vi "All together marble sorter code - working version 4_15.vi"() -> ()   [LabVIEW 2016]
uses:
  <vilib>/NXT/Block Support/NXT_InputPort.ctl
  <vilib>/NXT/Block Support/NXT_OutputPort.ctl
  <vilib>/NXT/Dual Mode Library/Sensors/Touch_Bumped.vi
  <vilib>/NXT/NXTIO Xnodes/NXTIONodeSubVIs/NXTMotorRunDistance.vi
  <vilib>/NXT/NXTIO Xnodes/NXTIONodeSubVIs/LEGOMoveAllMotorsDistance.vi
  <vilib>/NXT/Dual Mode Library/Sensors/Touch_Count.vi
  <vilib>/NXT/Dual Mode Library/Sensors/EV3_Color_Reflect.vi
  <vilib>/NXT/NXTIO Xnodes/NXTIONodeSubVIs/NXTStopMotors.vi
  <vilib>/NXT/NXTIO Xnodes/AddressXNode/NXTIOAddress.xnode
  <vilib>/NXT/NXTIO Xnodes/NXTIOXNode/NXTIO.xnode
  <vilib>/NXT/Subs/LVHSConnector.ctl
  <vilib>/NXT/LegoClasses/BrickReference/BrickReference.lvclass
panel:
  out "Marble Type 5":string
  out "Type 1 count 4":string
  out "Type 2 Count 4":string
  out "Marble Type 4 Code":i32[](array[numeric])
  out "Marble Count 4 Code":i32[](array[numeric])
  out "Marble Type 4":string
  out "Type 1 Count 3":string
  out "Type 2 Count 3":string
  out "Marble Count 3":i32[](array[numeric])
  out "Marble Type 3":i32[](array[numeric])
  out "Marble Type 2":string
  out "Type 1 Count 2":string
  out "Type 2 Count 2":string
  out "Marble Count 2 Code":i32[](array[numeric])
  out "Marble Type 2 Code":i32[](array[numeric])
  out "Marble Type code":i32[](array[numeric])
  out "Marble Size code":i32[](array[numeric])
  out "Marble Type":string
  out "Type 2 Count":string
  out "Type 1 Count":string
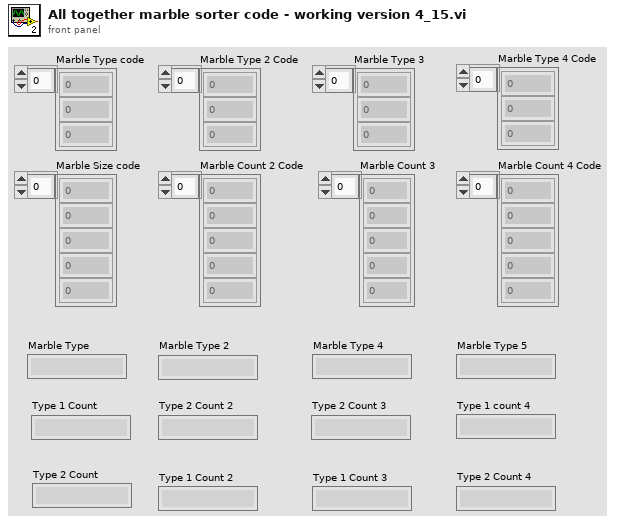
[diagram p1: front panel]
types:
  T1 = typedef "NXT_InputPort.ctl" = u32
  T2 = typedef "LVHSConnector.ctl" = refnum<class "BrickReference.lvclass">
  T3 = typedef "NXT_OutputPort.ctl" = u8
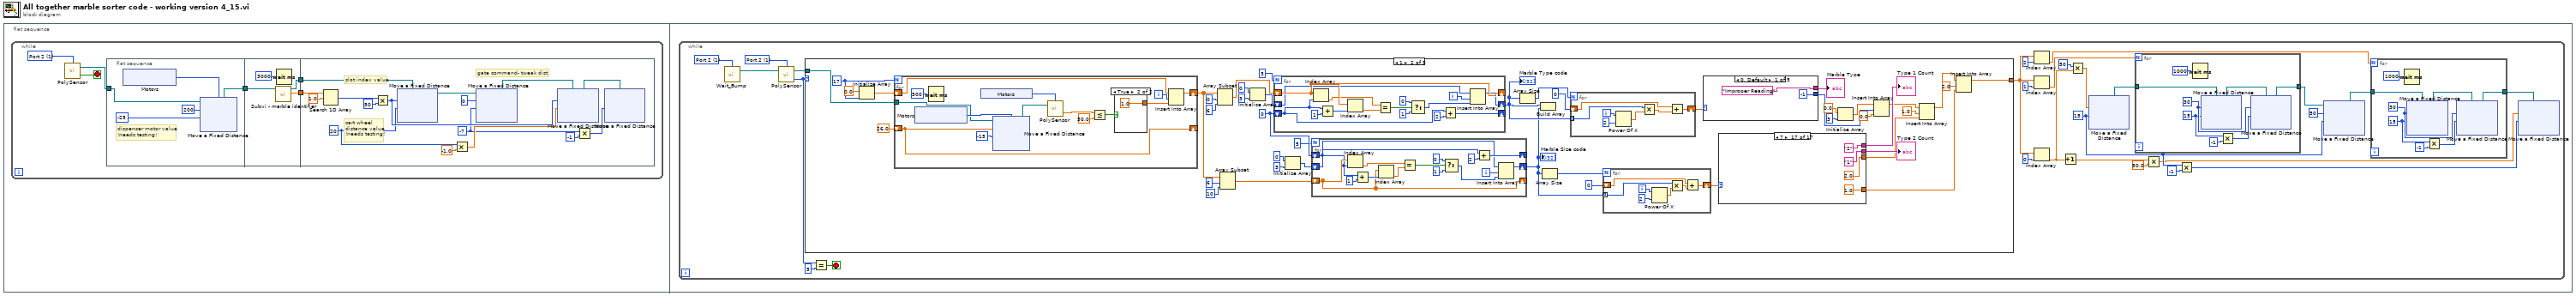
[diagram p0: block diagram]
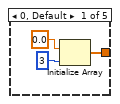
[diagram p2: hidden frame]
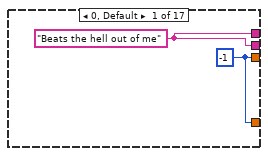
[diagram p3: hidden frame]
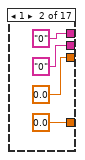
[diagram p4: hidden frame]
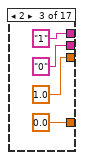
[diagram p5: hidden frame]
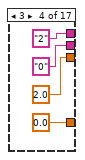
[diagram p6: hidden frame]
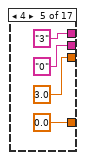
[diagram p7: hidden frame]
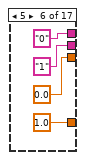
[diagram p8: hidden frame]
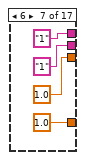
[diagram p9: hidden frame]
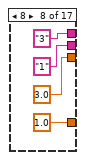
[diagram p10: hidden frame]
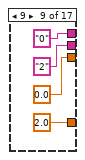
[diagram p11: hidden frame]
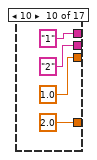
[diagram p12: hidden frame]
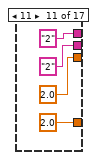
[diagram p13: hidden frame]
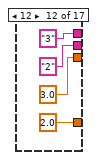
[diagram p14: hidden frame]
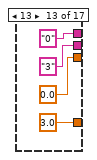
[diagram p15: hidden frame]
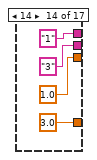
[diagram p16: hidden frame]
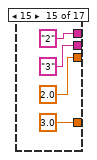
[diagram p17: hidden frame]
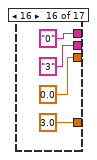
[diagram p18: hidden frame]
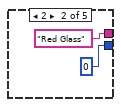
[diagram p19: hidden frame]
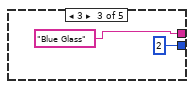
[diagram p20: hidden frame]
diagram:
  n1 = flat-sequence {
    frame #0 {
      n2 = while {
        stop <- w3 stop-if-true
        w1 = T1 1 items=["Port 1", "Port 2", "Port 3", "Port 4"] ("Port (Port 1)")
        n3 = call-poly <vilib>:"PolySensor.vi"("Port (Port 1)"=w1) -> ("Yes / No"=w3:bool, "NXT/EV3"=w2:T2)  [unwired: 2 in]
        n4 = flat-sequence {
          tunnel: [w8] -> w5
          tunnel: w2 -> [w7]
          tunnel: [w25] -> w6
          tunnel: w5 -> [w26]
          tunnel: [w24] -> w4
          tunnel: w6 -> [w37]
          tunnel: w4 -> [w28]
          frame #0 {
            # "dispenser motor value\n!needs testing!"
            n5 = xnode "Motors"() -> ("Motor"=w11:T3)
            n6 = xnode "Move a Fixed Distance"("Speed 1"=-25, "Distance 1"=200, "Motors"=w11, "NXT/EV3"=w7) -> ("NXT/EV3"=w8:T2)
          }
          frame #1 {
            n7 = call "Subvi - marble identifier.vi"("BrickReference in"=w26) -> ("Array"=w24:dbl[], "BrickReference out"=w25:T2)  [unwired: 9 in]
            n8 = Wait (ms)(milliseconds to wait=u32 3000) -> ()  [unwired: 1 out]
          }
          frame #2 {
            w30 = i8 -7 ("Speed 1")
            w39 = i8 20 ("Speed 1")
            # "gate command- tweak dist"
            # "cart wheel\ndistance value\n!needs testing!"
            # "slot index value"
            n9 = Search 1D Array(1D array=w28, element=1.0) -> (index of element=w27:i32)  [unwired: 1 in]
            n10 = Multiply(x=w27, y=50) -> (x*y=w41:i32)
            n11 = xnode "Move a Fixed Distance"("Speed 1"=w39, "Distance 1"=w41, "NXT/EV3"=w37) -> ("NXT/EV3"=w36:T2)  [unwired: 1 in]
            n12 = Multiply(x=w39, y=-1.0) -> (x*y=w38:dbl)
            n13 = xnode "Move a Fixed Distance"("Speed 1"=w30, "Distance 1"=0, "NXT/EV3"=w36) -> ("NXT/EV3"=w35:T2)  [unwired: 1 in]
            n14 = xnode "Move a Fixed Distance"("Speed 1"=w38, "Distance 1"=w41, "NXT/EV3"=w35) -> ("NXT/EV3"=w34:T2)  [unwired: 1 in]
            n15 = Multiply(x=w30, y=-1) -> (x*y=w31:i32)
            n16 = xnode "Move a Fixed Distance"("Speed 1"=w31, "NXT/EV3"=w34) -> ()  [unwired: 2 in, 1 out]
          }
        }
      }
    }
    frame #1 {
      n17 = while {
        stop <- w92 stop-if-true
        w77 = i8 15 ("Speed 1")
        w94 = T1 1 items=["Port 1", "Port 2", "Port 3", "Port 4"] ("Port (Port 1)")
        w95 = T1 1 items=["Port 1", "Port 2", "Port 3", "Port 4"] ("Port (Port 1)")
        n18 = call <vilib>:"Wait_Bump.vi"("Port (Port 1)"=w95) -> ("NXT/EV3"=w97:T2)  [unwired: 3 in]
        n19 = call-poly <vilib>:"PolySensor.vi"("NXT/EV3"=w97, "Port (Port 1)"=w94) -> ("Count"=w91:i16, "NXT/EV3"=w96:T2)  [unwired: 1 in]
        n20 = case shown="1" w91 {
          tunnel: w96 -> [_ w178 w375 w567 w766]
          tunnel: [w163 w166 w358 w550 w749] -> w81
          frame 0, Default {
            n21 = Initialize Array(0.0 ("element"), 3 ("dimension size")) -> (w163:dbl[])
          }
          frame 1 {
            w192 = 0
            w209 = 17
            n22 = Initialize Array(0.0, w209) -> (w207:dbl[])
            n23 = for {
              N: w209 -> [_]
              shift-right: [w338] -> w184
              shift-left: w207 -> [w342]
              shift-right: [w335] -> _
              shift-left: 26.0 -> [w335]
              tunnel: w178 -> [w330]
              i -> [w343]
              n24 = xnode "Motors"() -> ("Motor"=w333:T3)
              n25 = Wait (ms)(milliseconds to wait=500) -> ()  [unwired: 1 out]
              n26 = xnode "Motors"() -> ("Sensor"=w337:T1)
              n27 = xnode "Move a Fixed Distance"("Speed 1"=i8 -15, "Distance 1"=w335, "Motors"=w333, "NXT/EV3"=w330) -> ("NXT/EV3"=w334:T2)
              n28 = call-poly <vilib>:"PolySensor.vi"("NXT/EV3"=w334, "Port (Port 1)"=w337) -> ("Scaled Value"=w336:sgl)  [unwired: 1 in, 1 out]
              n29 = Less Or Equal?(x=w336, y=50.0) -> (x <= y?=w340:bool)
              n30 = case shown="True" w340 {
                tunnel: [0.0 1.0] -> w339
                frame False {
                }
                frame True {
                }
              }
              n31 = Insert Into Array(array=w342, index=w343, new element=w339) -> (w338:dbl[])
            }
            n32 = Array Subset(array=w184, index=0, length=6) -> (w200:dbl[])
            n33 = Array Subset(array=w184, index=6, length=10) -> (w196:dbl[])
            n34 = Initialize Array(0, 3 ("dimension size")) -> (w198:i32[])
            n35 = for {
              N: 3 -> [_]
              shift-right: [w327] -> _
              shift-left: w200 -> [w327]
              shift-right: [w319] -> _
              shift-left: w192 -> [w320]
              shift-right: [w317] -> w183
              shift-left: w198 -> [w316]
              i -> [w315]
              n36 = Index Array(array=w327, index=w320) -> (element=w324:dbl)
              n37 = Add(x=w320, y=1) -> (x+y=w328:i32)
              n38 = Index Array(array=w327, index=w328) -> (element=w323:dbl)
              n39 = Equal?(x=w324, y=w323) -> (x = y?=w322:bool)
              n40 = Select(t=0, s=w322, f=1) -> (s? t:f=w321:i32)
              n41 = Add(x=w320, y=2) -> (x+y=w319:i32)
              n42 = Insert Into Array(array=w316, index=w315, new element=w321) -> (w317:i32[])
            }
            "Marble Type code" <- w183
            n43 = Initialize Array(0, 5 ("dimension size")) -> (w193:i32[])
            n44 = for {
              N: 5 -> [_]
              shift-right: [w312] -> _
              shift-left: w196 -> [w312]
              shift-right: [w304] -> _
              shift-left: w192 -> [w305]
              shift-right: [w302] -> w182
              shift-left: w193 -> [w301]
              i -> [w300]
              n45 = Index Array(array=w312, index=w305) -> (element=w309:dbl)
              n46 = Add(x=w305, y=1) -> (x+y=w313:i32)
              n47 = Index Array(array=w312, index=w313) -> (element=w308:dbl)
              n48 = Equal?(x=w309, y=w308) -> (x = y?=w307:bool)
              n49 = Select(t=0, s=w307, f=1) -> (s? t:f=w306:i32)
              n50 = Add(x=w305, y=2) -> (x+y=w304:i32)
              n51 = Insert Into Array(array=w301, index=w300, new element=w306) -> (w302:i32[])
            }
            "Marble Size code" <- w182
            n52 = Array Size(array=w183) -> (size(s)=w190:i32)
            n53 = Build Array(w183, w182) -> ()  [unwired: 1 out]
            n54 = Array Size(array=w182) -> (size(s)=w187:i32)
            n55 = for {
              N: w190 -> [_]
              tunnel: w183 -> [w220] mode=indexing
              shift-right: [w217] -> w188
              shift-left: 0 -> [w218]
              i -> [w222]
              n56 = Power Of X(1:2, 2:w222) -> (0:w221:dbl)
              n57 = Multiply(x=w220, y=w221) -> (x*y=w219:dbl)
              n58 = Add(x=w218, y=w219) -> (x+y=w217:dbl)
            }
            n59 = for {
              N: w187 -> [_]
              tunnel: w182 -> [w213] mode=indexing
              shift-right: [w210] -> w185
              shift-left: 0 -> [w211]
              i -> [w215]
              n60 = Power Of X(1:2, 2:w215) -> (0:w214:dbl)
              n61 = Multiply(x=w213, y=w214) -> (x*y=w212:dbl)
              n62 = Add(x=w211, y=w212) -> (x+y=w210:dbl)
            }
            n63 = case shown="0, Default" w188 {
              tunnel: ["Improper Reading" "Red Glass" "Blue Glass" "White Glass" "Steel/HDPE"] -> w179
              tunnel: [-1 0 2 4 6] -> w169
              frame 0, Default {
              }
              frame 2 {
              }
              frame 3 {
              }
              frame 1 {
              }
              frame 4 {
              }
            }
            "Marble Type" <- w179
            n64 = case shown="7" w185 {
              tunnel: [w225 "0" "1" "2" "3" "0" "1" "3" "0" "1" "2" "3" "0" "1" "2" "0" "2"] -> w181
              tunnel: [w225 "0" "0" "0" "0" "1" "1" "1" "2" "2" "2" "2" "3" "3" "3" "3" "1"] -> w180
              tunnel: [w224 0.0 ("new element/subarray") 1.0 ("new element/subarray") 2.0 ("new element/subarray") 3.0 ("new element/subarray") 0.0 ("new element/subarray") 1.0 ("new element/subarray") 3.0 ("new element/subarray") 0.0 ("new element/subarray") 1.0 ("new element/subarray") 2.0 ("new element/subarray") 3.0 ("new element/subarray") 0.0 ("new element/subarray") 1.0 ("new element/subarray") 2.0 ("new element/subarray") 0.0 ("new element/subarray") 2.0 ("new element/subarray")] -> w168
              tunnel: [w224 0.0 ("new element/subarray") 0.0 ("new element/subarray") 0.0 ("new element/subarray") 0.0 ("new element/subarray") 1.0 ("new element/subarray") 1.0 ("new element/subarray") 1.0 ("new element/subarray") 2.0 ("new element/subarray") 2.0 ("new element/subarray") 2.0 ("new element/subarray") 2.0 ("new element/subarray") 3.0 ("new element/subarray") 3.0 ("new element/subarray") 3.0 ("new element/subarray") 3.0 ("new element/subarray") 1.0 ("new element/subarray")] -> w167
              frame 0, Default {
                w224 = -1
                w225 = "Beats the hell out of me"
              }
              frame 1 {
              }
              frame 2 {
              }
              frame 3 {
              }
              frame 4 {
              }
              frame 5 {
              }
              frame 6 {
              }
              frame 8 {
              }
              frame 9 {
              }
              frame 10 {
              }
              frame 11 {
              }
              frame 12 {
              }
              frame 13 {
              }
              frame 14 {
              }
              frame 15 {
              }
              frame 16 {
              }
              frame 7 {
              }
            }
            "Type 2 Count" <- w180
            "Type 1 Count" <- w181
            n65 = Initialize Array(0.0 ("element"), 3 ("dimension size")) -> (w175:dbl[])
            n66 = Insert Into Array(array=w175, index=w169, new element=0.0 ("new element/subarray")) -> (w174:dbl[])
            n67 = Insert Into Array(array=w174, index=1.0 ("new element/subarray"), new element=w168) -> (w173:dbl[])
            n68 = Insert Into Array(array=w173, index=2.0 ("new element/subarray"), new element=w167) -> (w166:dbl[])
          }
          frame 2 {
            w384 = 0
            w401 = 17
            n69 = Initialize Array(0.0, w401) -> (w399:dbl[])
            n70 = for {
              N: w401 -> [_]
              shift-right: [w530] -> w378
              shift-left: w399 -> [w534]
              shift-right: [w527] -> _
              shift-left: 26.0 -> [w527]
              tunnel: w375 -> [w522]
              i -> [w535]
              n71 = xnode "Motors"() -> ("Motor"=w525:T3)
              n72 = Wait (ms)(milliseconds to wait=500) -> ()  [unwired: 1 out]
              n73 = xnode "Motors"() -> ("Sensor"=w529:T1)
              n74 = xnode "Move a Fixed Distance"("Speed 1"=i8 -15, "Distance 1"=w527, "Motors"=w525, "NXT/EV3"=w522) -> ("NXT/EV3"=w526:T2)
              n75 = call-poly <vilib>:"PolySensor.vi"("NXT/EV3"=w526, "Port (Port 1)"=w529) -> ("Scaled Value"=w528:sgl)  [unwired: 1 in, 1 out]
              n76 = Less Or Equal?(x=w528, y=50.0) -> (x <= y?=w532:bool)
              n77 = case shown="True" w532 {
                tunnel: [0.0 1.0] -> w531
                frame False {
                }
                frame True {
                }
              }
              n78 = Insert Into Array(array=w534, index=w535, new element=w531) -> (w530:dbl[])
            }
            n79 = Array Subset(array=w378, index=0, length=6) -> (w392:dbl[])
            n80 = Array Subset(array=w378, index=6, length=10) -> (w388:dbl[])
            n81 = Initialize Array(0, 3 ("dimension size")) -> (w390:i32[])
            n82 = for {
              N: 3 -> [_]
              shift-right: [w519] -> _
              shift-left: w392 -> [w519]
              shift-right: [w511] -> _
              shift-left: w384 -> [w512]
              shift-right: [w509] -> w377
              shift-left: w390 -> [w508]
              i -> [w507]
              n83 = Index Array(array=w519, index=w512) -> (element=w516:dbl)
              n84 = Add(x=w512, y=1) -> (x+y=w520:i32)
              n85 = Index Array(array=w519, index=w520) -> (element=w515:dbl)
              n86 = Equal?(x=w516, y=w515) -> (x = y?=w514:bool)
              n87 = Select(t=0, s=w514, f=1) -> (s? t:f=w513:i32)
              n88 = Add(x=w512, y=2) -> (x+y=w511:i32)
              n89 = Insert Into Array(array=w508, index=w507, new element=w513) -> (w509:i32[])
            }
            "Marble Type 2 Code" <- w377
            n90 = Initialize Array(0, 5 ("dimension size")) -> (w385:i32[])
            n91 = for {
              N: 5 -> [_]
              shift-right: [w504] -> _
              shift-left: w388 -> [w504]
              shift-right: [w496] -> _
              shift-left: w384 -> [w497]
              shift-right: [w494] -> w376
              shift-left: w385 -> [w493]
              i -> [w492]
              n92 = Index Array(array=w504, index=w497) -> (element=w501:dbl)
              n93 = Add(x=w497, y=1) -> (x+y=w505:i32)
              n94 = Index Array(array=w504, index=w505) -> (element=w500:dbl)
              n95 = Equal?(x=w501, y=w500) -> (x = y?=w499:bool)
              n96 = Select(t=0, s=w499, f=1) -> (s? t:f=w498:i32)
              n97 = Add(x=w497, y=2) -> (x+y=w496:i32)
              n98 = Insert Into Array(array=w493, index=w492, new element=w498) -> (w494:i32[])
            }
            "Marble Count 2 Code" <- w376
            n99 = Array Size(array=w377) -> (size(s)=w382:i32)
            n100 = Array Size(array=w376) -> (size(s)=w380:i32)
            n101 = for {
              N: w382 -> [_]
              tunnel: w377 -> [w488] mode=indexing
              shift-right: [w485] -> w361
              shift-left: 0 -> [w486]
              i -> [w490]
              n102 = Power Of X(1:2, 2:w490) -> (0:w489:dbl)
              n103 = Multiply(x=w488, y=w489) -> (x*y=w487:dbl)
              n104 = Add(x=w486, y=w487) -> (x+y=w485:dbl)
            }
            n105 = for {
              N: w380 -> [_]
              tunnel: w376 -> [w481] mode=indexing
              shift-right: [w478] -> w359
              shift-left: 0 -> [w479]
              i -> [w483]
              n106 = Power Of X(1:2, 2:w483) -> (0:w482:dbl)
              n107 = Multiply(x=w481, y=w482) -> (x*y=w480:dbl)
              n108 = Add(x=w479, y=w480) -> (x+y=w478:dbl)
            }
            n109 = case shown="0, Default" w361 {
              tunnel: ["Improper Reading" "Red Glass" "Blue Glass" "White Glass" "Steel/HDPE"] -> w362
              tunnel: [-1 0 2 4 6] -> w360
              frame 0, Default {
              }
              frame 2 {
              }
              frame 3 {
              }
              frame 1 {
              }
              frame 4 {
              }
            }
            "Marble Type 2" <- w362
            n110 = case shown="7" w359 {
              tunnel: [w403 "0" "1" "2" "3" "0" "1" "3" "0" "1" "2" "3" "0" "1" "2" "0" "2"] -> w364
              tunnel: [w403 "0" "0" "0" "0" "1" "1" "1" "2" "2" "2" "2" "3" "3" "3" "3" "1"] -> w363
              tunnel: [w402 0.0 ("new element/subarray") 1.0 ("new element/subarray") 2.0 ("new element/subarray") 3.0 ("new element/subarray") 0.0 ("new element/subarray") 1.0 ("new element/subarray") 3.0 ("new element/subarray") 0.0 ("new element/subarray") 1.0 ("new element/subarray") 2.0 ("new element/subarray") 3.0 ("new element/subarray") 0.0 ("new element/subarray") 1.0 ("new element/subarray") 2.0 ("new element/subarray") 0.0 ("new element/subarray") 2.0 ("new element/subarray")] -> w366
              tunnel: [w402 0.0 ("new element/subarray") 0.0 ("new element/subarray") 0.0 ("new element/subarray") 0.0 ("new element/subarray") 1.0 ("new element/subarray") 1.0 ("new element/subarray") 1.0 ("new element/subarray") 2.0 ("new element/subarray") 2.0 ("new element/subarray") 2.0 ("new element/subarray") 2.0 ("new element/subarray") 3.0 ("new element/subarray") 3.0 ("new element/subarray") 3.0 ("new element/subarray") 3.0 ("new element/subarray") 1.0 ("new element/subarray")] -> w365
              frame 0, Default {
                w402 = -1
                w403 = "Beats the hell out of me"
              }
              frame 1 {
              }
              frame 2 {
              }
              frame 3 {
              }
              frame 4 {
              }
              frame 5 {
              }
              frame 6 {
              }
              frame 8 {
              }
              frame 9 {
              }
              frame 10 {
              }
              frame 11 {
              }
              frame 12 {
              }
              frame 13 {
              }
              frame 14 {
              }
              frame 15 {
              }
              frame 16 {
              }
              frame 7 {
              }
            }
            "Type 1 Count 2" <- w364
            "Type 2 Count 2" <- w363
            n111 = Initialize Array(0.0 ("element"), 3 ("dimension size")) -> (w372:dbl[])
            n112 = Insert Into Array(array=w372, index=w360, new element=0.0 ("new element/subarray")) -> (w371:dbl[])
            n113 = Insert Into Array(array=w371, index=1.0 ("new element/subarray"), new element=w366) -> (w370:dbl[])
            n114 = Insert Into Array(array=w370, index=2.0 ("new element/subarray"), new element=w365) -> (w358:dbl[])
          }
          frame 3 {
            w586 = 0
            w569 = 17
            n115 = Initialize Array(0.0, w569) -> (w571:dbl[])
            n116 = for {
              N: w569 -> [_]
              shift-right: [w723] -> w592
              shift-left: w571 -> [w727]
              shift-right: [w720] -> _
              shift-left: 26.0 -> [w720]
              tunnel: w567 -> [w714]
              i -> [w728]
              n117 = xnode "Motors"() -> ("Motor"=w715:T3)
              n118 = xnode "Motors"() -> ("Motor"=w718:T3)
              n119 = Wait (ms)(milliseconds to wait=500) -> ()  [unwired: 1 out]
              n120 = xnode "Stop Motors"("Motors"=w715) -> ()  [unwired: 1 in, 1 out]
              n121 = xnode "Motors"() -> ("Sensor"=w722:T1)
              n122 = xnode "Move a Fixed Distance"("Speed 1"=i8 -15, "Distance 1"=w720, "Motors"=w718, "NXT/EV3"=w714) -> ("NXT/EV3"=w719:T2)
              n123 = call-poly <vilib>:"PolySensor.vi"("NXT/EV3"=w719, "Port (Port 1)"=w722) -> ("Scaled Value"=w721:sgl)  [unwired: 1 in, 1 out]
              n124 = Less Or Equal?(x=w721, y=50.0) -> (x <= y?=w725:bool)
              n125 = case shown="True" w725 {
                tunnel: [0.0 1.0] -> w724
                frame False {
                }
                frame True {
                }
              }
              n126 = Insert Into Array(array=w727, index=w728, new element=w724) -> (w723:dbl[])
            }
            n127 = Array Subset(array=w592, index=0, length=6) -> (w578:dbl[])
            n128 = Array Subset(array=w592, index=6, length=10) -> (w582:dbl[])
            n129 = Initialize Array(0, 3 ("dimension size")) -> (w580:i32[])
            n130 = for {
              N: 3 -> [_]
              shift-right: [w711] -> _
              shift-left: w578 -> [w711]
              shift-right: [w703] -> _
              shift-left: w586 -> [w704]
              shift-right: [w701] -> w593
              shift-left: w580 -> [w700]
              i -> [w699]
              n131 = Index Array(array=w711, index=w704) -> (element=w708:dbl)
              n132 = Add(x=w704, y=1) -> (x+y=w712:i32)
              n133 = Index Array(array=w711, index=w712) -> (element=w707:dbl)
              n134 = Equal?(x=w708, y=w707) -> (x = y?=w706:bool)
              n135 = Select(t=0, s=w706, f=1) -> (s? t:f=w705:i32)
              n136 = Add(x=w704, y=2) -> (x+y=w703:i32)
              n137 = Insert Into Array(array=w700, index=w699, new element=w705) -> (w701:i32[])
            }
            "Marble Type 3" <- w593
            n138 = Initialize Array(0, 5 ("dimension size")) -> (w585:i32[])
            n139 = for {
              N: 5 -> [_]
              shift-right: [w696] -> _
              shift-left: w582 -> [w696]
              shift-right: [w688] -> _
              shift-left: w586 -> [w689]
              shift-right: [w686] -> w568
              shift-left: w585 -> [w685]
              i -> [w684]
              n140 = Index Array(array=w696, index=w689) -> (element=w693:dbl)
              n141 = Add(x=w689, y=1) -> (x+y=w697:i32)
              n142 = Index Array(array=w696, index=w697) -> (element=w692:dbl)
              n143 = Equal?(x=w693, y=w692) -> (x = y?=w691:bool)
              n144 = Select(t=0, s=w691, f=1) -> (s? t:f=w690:i32)
              n145 = Add(x=w689, y=2) -> (x+y=w688:i32)
              n146 = Insert Into Array(array=w685, index=w684, new element=w690) -> (w686:i32[])
            }
            "Marble Count 3" <- w568
            n147 = Array Size(array=w593) -> (size(s)=w588:i32)
            n148 = Array Size(array=w568) -> (size(s)=w590:i32)
            n149 = for {
              N: w588 -> [_]
              tunnel: w593 -> [w680] mode=indexing
              shift-right: [w677] -> w551
              shift-left: 0 -> [w678]
              i -> [w682]
              n150 = Power Of X(1:2, 2:w682) -> (0:w681:dbl)
              n151 = Multiply(x=w680, y=w681) -> (x*y=w679:dbl)
              n152 = Add(x=w678, y=w679) -> (x+y=w677:dbl)
            }
            n153 = for {
              N: w590 -> [_]
              tunnel: w568 -> [w673] mode=indexing
              shift-right: [w670] -> w552
              shift-left: 0 -> [w671]
              i -> [w675]
              n154 = Power Of X(1:2, 2:w675) -> (0:w674:dbl)
              n155 = Multiply(x=w673, y=w674) -> (x*y=w672:dbl)
              n156 = Add(x=w671, y=w672) -> (x+y=w670:dbl)
            }
            n157 = case shown="0, Default" w551 {
              tunnel: ["Improper Reading" "Red Glass" "Blue Glass" "White Glass" "Steel/HDPE"] -> w556
              tunnel: [-1 0 2 4 6] -> w553
              frame 0, Default {
              }
              frame 2 {
              }
              frame 3 {
              }
              frame 1 {
              }
              frame 4 {
              }
            }
            "Marble Type 4" <- w556
            n158 = case shown="7" w552 {
              tunnel: [w595 "0" "1" "2" "3" "0" "1" "3" "0" "1" "2" "3" "0" "1" "2" "0" "2"] -> w555
              tunnel: [w595 "0" "0" "0" "0" "1" "1" "1" "2" "2" "2" "2" "3" "3" "3" "3" "1"] -> w554
              tunnel: [w594 0.0 ("new element/subarray") 1.0 ("new element/subarray") 2.0 ("new element/subarray") 3.0 ("new element/subarray") 0.0 ("new element/subarray") 1.0 ("new element/subarray") 3.0 ("new element/subarray") 0.0 ("new element/subarray") 1.0 ("new element/subarray") 2.0 ("new element/subarray") 3.0 ("new element/subarray") 0.0 ("new element/subarray") 1.0 ("new element/subarray") 2.0 ("new element/subarray") 0.0 ("new element/subarray") 2.0 ("new element/subarray")] -> w558
              tunnel: [w594 0.0 ("new element/subarray") 0.0 ("new element/subarray") 0.0 ("new element/subarray") 0.0 ("new element/subarray") 1.0 ("new element/subarray") 1.0 ("new element/subarray") 1.0 ("new element/subarray") 2.0 ("new element/subarray") 2.0 ("new element/subarray") 2.0 ("new element/subarray") 2.0 ("new element/subarray") 3.0 ("new element/subarray") 3.0 ("new element/subarray") 3.0 ("new element/subarray") 3.0 ("new element/subarray") 1.0 ("new element/subarray")] -> w557
              frame 0, Default {
                w594 = -1
                w595 = "Beats the hell out of me"
              }
              frame 1 {
              }
              frame 2 {
              }
              frame 3 {
              }
              frame 4 {
              }
              frame 5 {
              }
              frame 6 {
              }
              frame 8 {
              }
              frame 9 {
              }
              frame 10 {
              }
              frame 11 {
              }
              frame 12 {
              }
              frame 13 {
              }
              frame 14 {
              }
              frame 15 {
              }
              frame 16 {
              }
              frame 7 {
              }
            }
            "Type 1 Count 3" <- w555
            "Type 2 Count 3" <- w554
            n159 = Initialize Array(0.0 ("element"), 3 ("dimension size")) -> (w564:dbl[])
            n160 = Insert Into Array(array=w564, index=w553, new element=0.0 ("new element/subarray")) -> (w563:dbl[])
            n161 = Insert Into Array(array=w563, index=1.0 ("new element/subarray"), new element=w558) -> (w562:dbl[])
            n162 = Insert Into Array(array=w562, index=2.0 ("new element/subarray"), new element=w557) -> (w550:dbl[])
          }
          frame 4 {
            w784 = 0
            w767 = 17
            n163 = Initialize Array(0.0, w767) -> (w769:dbl[])
            n164 = for {
              N: w767 -> [_]
              shift-right: [w924] -> w790
              shift-left: w769 -> [w928]
              shift-right: [w921] -> _
              shift-left: 26.0 -> [w921]
              tunnel: w766 -> [w915]
              tunnel: [w913] -> _
              i -> [w929]
              n165 = xnode "Motors"() -> ("Motor"=w919:T3)
              n166 = Wait (ms)(milliseconds to wait=500) -> ()  [unwired: 1 out]
              n167 = xnode "Motors"() -> ("Sensor"=w923:T1)
              n168 = xnode "Move a Fixed Distance"("Speed 1"=i8 -15, "Distance 1"=w921, "Motors"=w919, "NXT/EV3"=w915) -> ("NXT/EV3"=w920:T2)
              n169 = xnode "Motors"() -> ("Motor"=w916:T3)
              n170 = call-poly <vilib>:"PolySensor.vi"("NXT/EV3"=w920, "Port (Port 1)"=w923) -> ("Scaled Value"=w922:sgl, "NXT/EV3"=w914:T2)  [unwired: 1 in]
              n171 = xnode "Stop Motors"("Motors"=w916, "NXT/EV3"=w914) -> ("NXT/EV3"=w913:T2)
              n172 = Less Or Equal?(x=w922, y=50.0) -> (x <= y?=w926:bool)
              n173 = case shown="True" w926 {
                tunnel: [0.0 1.0] -> w925
                frame False {
                }
                frame True {
                }
              }
              n174 = Insert Into Array(array=w928, index=w929, new element=w925) -> (w924:dbl[])
            }
            n175 = Array Subset(array=w790, index=0, length=6) -> (w776:dbl[])
            n176 = Array Subset(array=w790, index=6, length=10) -> (w780:dbl[])
            n177 = Initialize Array(0, 3 ("dimension size")) -> (w778:i32[])
            n178 = for {
              N: 3 -> [_]
              shift-right: [w910] -> _
              shift-left: w776 -> [w910]
              shift-right: [w902] -> _
              shift-left: w784 -> [w903]
              shift-right: [w900] -> w791
              shift-left: w778 -> [w899]
              i -> [w898]
              n179 = Index Array(array=w910, index=w903) -> (element=w907:dbl)
              n180 = Add(x=w903, y=1) -> (x+y=w911:i32)
              n181 = Index Array(array=w910, index=w911) -> (element=w906:dbl)
              n182 = Equal?(x=w907, y=w906) -> (x = y?=w905:bool)
              n183 = Select(t=0, s=w905, f=1) -> (s? t:f=w904:i32)
              n184 = Add(x=w903, y=2) -> (x+y=w902:i32)
              n185 = Insert Into Array(array=w899, index=w898, new element=w904) -> (w900:i32[])
            }
            "Marble Type 4 Code" <- w791
            n186 = Initialize Array(0, 5 ("dimension size")) -> (w783:i32[])
            n187 = for {
              N: 5 -> [_]
              shift-right: [w895] -> _
              shift-left: w780 -> [w895]
              shift-right: [w887] -> _
              shift-left: w784 -> [w888]
              shift-right: [w885] -> w792
              shift-left: w783 -> [w884]
              i -> [w883]
              n188 = Index Array(array=w895, index=w888) -> (element=w892:dbl)
              n189 = Add(x=w888, y=1) -> (x+y=w896:i32)
              n190 = Index Array(array=w895, index=w896) -> (element=w891:dbl)
              n191 = Equal?(x=w892, y=w891) -> (x = y?=w890:bool)
              n192 = Select(t=0, s=w890, f=1) -> (s? t:f=w889:i32)
              n193 = Add(x=w888, y=2) -> (x+y=w887:i32)
              n194 = Insert Into Array(array=w884, index=w883, new element=w889) -> (w885:i32[])
            }
            "Marble Count 4 Code" <- w792
            n195 = Array Size(array=w791) -> (size(s)=w786:i32)
            n196 = Array Size(array=w792) -> (size(s)=w788:i32)
            n197 = for {
              N: w786 -> [_]
              tunnel: w791 -> [w879] mode=indexing
              shift-right: [w876] -> w750
              shift-left: 0 -> [w877]
              i -> [w881]
              n198 = Power Of X(1:2, 2:w881) -> (0:w880:dbl)
              n199 = Multiply(x=w879, y=w880) -> (x*y=w878:dbl)
              n200 = Add(x=w877, y=w878) -> (x+y=w876:dbl)
            }
            n201 = for {
              N: w788 -> [_]
              tunnel: w792 -> [w872] mode=indexing
              shift-right: [w869] -> w751
              shift-left: 0 -> [w870]
              i -> [w874]
              n202 = Power Of X(1:2, 2:w874) -> (0:w873:dbl)
              n203 = Multiply(x=w872, y=w873) -> (x*y=w871:dbl)
              n204 = Add(x=w870, y=w871) -> (x+y=w869:dbl)
            }
            n205 = case shown="0, Default" w750 {
              tunnel: ["Improper Reading" "Red Glass" "Blue Glass" "White Glass" "Steel/HDPE"] -> w755
              tunnel: [-1 0 2 4 6] -> w752
              frame 0, Default {
              }
              frame 2 {
              }
              frame 3 {
              }
              frame 1 {
              }
              frame 4 {
              }
            }
            "Marble Type 5" <- w755
            n206 = case shown="7" w751 {
              tunnel: [w794 "0" "1" "2" "3" "0" "1" "3" "0" "1" "2" "3" "0" "1" "2" "0" "2"] -> w754
              tunnel: [w794 "0" "0" "0" "0" "1" "1" "1" "2" "2" "2" "2" "3" "3" "3" "3" "1"] -> w753
              tunnel: [w793 0.0 ("new element/subarray") 1.0 ("new element/subarray") 2.0 ("new element/subarray") 3.0 ("new element/subarray") 0.0 ("new element/subarray") 1.0 ("new element/subarray") 3.0 ("new element/subarray") 0.0 ("new element/subarray") 1.0 ("new element/subarray") 2.0 ("new element/subarray") 3.0 ("new element/subarray") 0.0 ("new element/subarray") 1.0 ("new element/subarray") 2.0 ("new element/subarray") 0.0 ("new element/subarray") 2.0 ("new element/subarray")] -> w757
              tunnel: [w793 0.0 ("new element/subarray") 0.0 ("new element/subarray") 0.0 ("new element/subarray") 0.0 ("new element/subarray") 1.0 ("new element/subarray") 1.0 ("new element/subarray") 1.0 ("new element/subarray") 2.0 ("new element/subarray") 2.0 ("new element/subarray") 2.0 ("new element/subarray") 2.0 ("new element/subarray") 3.0 ("new element/subarray") 3.0 ("new element/subarray") 3.0 ("new element/subarray") 3.0 ("new element/subarray") 1.0 ("new element/subarray")] -> w756
              frame 0, Default {
                w793 = -1
                w794 = "Beats the hell out of me"
              }
              frame 1 {
              }
              frame 2 {
              }
              frame 3 {
              }
              frame 4 {
              }
              frame 5 {
              }
              frame 6 {
              }
              frame 8 {
              }
              frame 9 {
              }
              frame 10 {
              }
              frame 11 {
              }
              frame 12 {
              }
              frame 13 {
              }
              frame 14 {
              }
              frame 15 {
              }
              frame 16 {
              }
              frame 7 {
              }
            }
            "Type 1 count 4" <- w754
            "Type 2 Count 4" <- w753
            n207 = Initialize Array(0.0 ("element"), 3 ("dimension size")) -> (w763:dbl[])
            n208 = Insert Into Array(array=w763, index=w752, new element=0.0 ("new element/subarray")) -> (w762:dbl[])
            n209 = Insert Into Array(array=w762, index=1.0 ("new element/subarray"), new element=w757) -> (w761:dbl[])
            n210 = Insert Into Array(array=w761, index=2.0 ("new element/subarray"), new element=w756) -> (w749:dbl[])
          }
        }
        n211 = Equal?(x=w91, y=5) -> (x = y?=w92:bool)
        n212 = Index Array(array=w81, index=2) -> (element=w79:dbl)
        n213 = Index Array(array=w81, index=1) -> (element=w85:dbl)
        n214 = Index Array(array=w81, index=0) -> (element=w75:dbl)
        n215 = Increment(x=w75) -> (x+1=w74:dbl)
        n216 = Multiply(x=50, y=w75) -> (x*y=w88:dbl)
        n217 = xnode "Move a Fixed Distance"("Speed 1"=w77, "Distance 1"=w88) -> ("NXT/EV3"=w87:T2)  [unwired: 2 in]
        n218 = for {
          N: w85 -> [_]
          tunnel: w87 -> [w141]
          tunnel: [w134] -> w84
          w139 = 30 ("Distance 1")
          w137 = i8 15 ("Speed 1")
          n219 = Wait (ms)(milliseconds to wait=u32 1000) -> ()  [unwired: 1 out]
          n220 = xnode "Move a Fixed Distance"("Speed 1"=w137, "Distance 1"=w139, "NXT/EV3"=w141) -> ("NXT/EV3"=w135:T2)  [unwired: 1 in]
          n221 = Multiply(x=w137, y=-1) -> (x*y=w136:i32)
          n222 = xnode "Move a Fixed Distance"("Speed 1"=w136, "Distance 1"=w139, "NXT/EV3"=w135) -> ("NXT/EV3"=w134:T2)  [unwired: 1 in]
        }
        n223 = Multiply(x=w74, y=50.0) -> (x*y=w72:dbl)
        n224 = Multiply(x=w77, y=-1) -> (x*y=w76:i32)
        n225 = xnode "Move a Fixed Distance"("Speed 1"=w77, "Distance 1"=50, "NXT/EV3"=w84) -> ("NXT/EV3"=w83:T2)  [unwired: 1 in]
        n226 = for {
          N: w79 -> [_]
          tunnel: w83 -> [w119]
          tunnel: [w112] -> w71
          w117 = 30 ("Distance 1")
          w115 = i8 15 ("Speed 1")
          n227 = Wait (ms)(milliseconds to wait=u32 1000) -> ()  [unwired: 1 out]
          n228 = xnode "Move a Fixed Distance"("Speed 1"=w115, "Distance 1"=w117, "NXT/EV3"=w119) -> ("NXT/EV3"=w113:T2)  [unwired: 1 in]
          n229 = Multiply(x=w115, y=-1) -> (x*y=w114:i32)
          n230 = xnode "Move a Fixed Distance"("Speed 1"=w114, "Distance 1"=w117, "NXT/EV3"=w113) -> ("NXT/EV3"=w112:T2)  [unwired: 1 in]
        }
        n231 = xnode "Move a Fixed Distance"("Speed 1"=w76, "Distance 1"=w72, "NXT/EV3"=w71) -> ()  [unwired: 1 in, 1 out]
      }
    }
  }
